vi "Helper Files_User Events.vi"() -> (3 "Init Dialog UEs":T1)   [LabVIEW 2023]
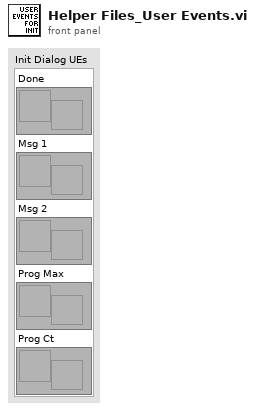
[diagram p1: front panel]
types:
  T1 = cluster{"Done":refnum<user-event>, "Msg 1":refnum<user-event>, "Msg 2":refnum<user-event>, "Prog Max":refnum<user-event>, "Prog Ct":refnum<user-event>}
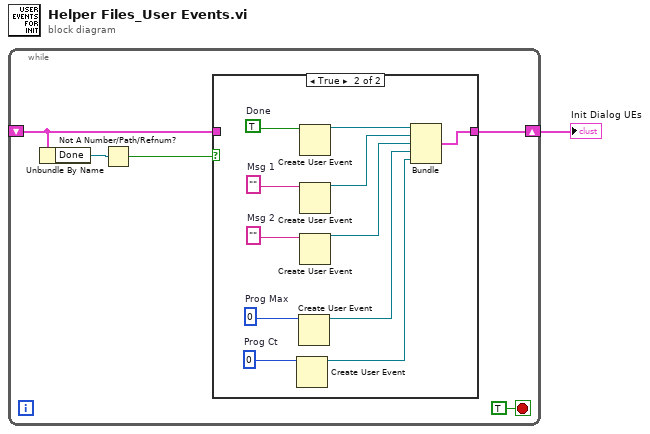
[diagram p0: block diagram]
diagram:
  n1 = while {
    shift-right: [w6] -> w1
    shift-left: _ -> [w2]
    stop <- TRUE stop-if-true
    n2 = Unbundle By Name(w2) -> ("Done"=w4:refnum<user-event>)
    n3 = Not A Number/Path/Refnum?(number/path/refnum=w4) -> (NaN/Path/Refnum?=w3:bool)
    n4 = case shown="True" w3 {
      tunnel: [w7 w14] -> w6
      tunnel: w2 -> [w7 _]
      frame False {
      }
      frame True {
        w9 = ""  # Msg 2
        w12 = u32 0  # Prog Ct
        w13 = u32 0  # Prog Max
        w17 = ""  # Msg 1
        w18 = TRUE  # Done
        n5 = Create User Event(user event datatype=w12) -> (user event=w10:refnum<user-event>)  [unwired: 1 in, 1 out]
        n6 = Create User Event(user event datatype=w13) -> (user event=w11:refnum<user-event>)  [unwired: 1 in, 1 out]
        n7 = Create User Event(user event datatype=w18) -> (user event=w16:refnum<user-event>)  [unwired: 1 in, 1 out]
        n8 = Create User Event(user event datatype=w17) -> (user event=w15:refnum<user-event>)  [unwired: 1 in, 1 out]
        n9 = Create User Event(user event datatype=w9) -> (user event=w8:refnum<user-event>)  [unwired: 1 in, 1 out]
        n10 = Bundle("Done"=w16, "Msg 1"=w15, "Msg 2"=w8, "Prog Max"=w11, "Prog Ct"=w10) -> (w14:T1)  [unwired: 1 in]
      }
    }
  }
  "Init Dialog UEs" <- w1
